vi "Finalize.vi"(8 "error in (no error)":errorcluster, 11 "SQL Statement in":refnum<class "SQL Statement.lvclass">) -> (0 "error out":errorcluster)   [LabVIEW 2013, in "SQLiteSupport.lvlib" / "SQL Statement.lvclass"]
doc: "Releases (destroys) a prepare SQL statement. \n\nThis VI will operate even if an error is input into the \"error in\" terminal. Unlike with the C interface \"sqlite3_finalize\" command, this VI does NOT return the error code of the previously executed \"step\"."
uses:
  SQL Statement.lvclass
  SQL Statement.lvclass/SQL Statement.ctl
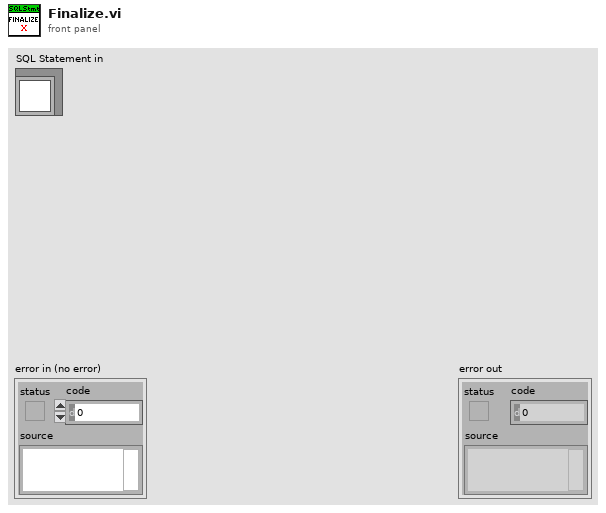
[diagram p1: front panel]
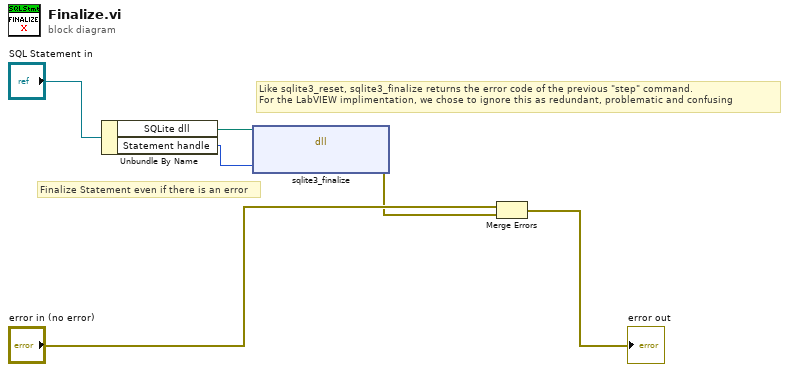
[diagram p0: block diagram]
diagram:
  # "Finalize Statement even if there is an error"
  # "Like sqlite3_reset, sqlite3_finalize returns the error code of the previous \"step\" command.\nFor the LabVIEW implimentation, we chose to ignore this as redundant, problematic and confusing"
  n1 = Unbundle By Name("SQL Statement in") -> ("SQLite dll"=w5:path, "Statement handle"=w4:u64)
  n2 = dll-call lib="C:/SQLite/sqlite3.dll" fn="sqlite3_finalize"(path in=w5, "Statement"=w4) -> (error out=w1:errorcluster)  [unwired: 4 in, 1 out]
  n3 = Merge Errors("error in (no error)", w1) -> (→"error out":errorcluster)
